vi "KI6221.vi"() -> ()   [LabVIEW 2019] (continued)
                n2609 = call "WriteToFile.vi"("character string"=w5028, "file path (dialog if empty)"=w4969) -> ("new file path (Not A Path if cancelled)"=w5027:path)  [unwired: 3 in]
                n2610 = Path To String(path=w5027) -> (string=w4971:string)
                n2611 = Equal?(x=w4972, y=w4971) -> (x = y?=w4970:bool)
                n2612 = call "CreateDataFiles.vi"("new file path (Not A Path if cancelled)"=w5025, "attachments"="attachments", "path"=w4969, "selection"=w4970, "DELTA DATASHEET"=w4974, "PULSE DATASHEET"=w4975, "DIFF CON DATASHEET"=w4976, "ATTACHMENTS"=w4977) -> ()
              }
              frame True {
              }
            }
          }
        }
        n2613 = control-ref of="Main Tabs"() -> (w156:refnum<vi>)
        n2614 = control-ref of="COMM\nTab Control"() -> (w189:refnum<vi>)
        n2615 = control-ref of="4 step TABS"() -> (w188:refnum<vi>)
        n2616 = control-ref of="Default path"() -> (w190:refnum<vi>)
        n2617 = local read "attachments"() -> (w186:T6)
        n2618 = local read "mail server"() -> (w187:string)
        n2619 = control-ref of="debug str"() -> (w173:refnum<vi>)
        n2620 = control-ref of="Main Tabs"() -> (w155:refnum<vi>)
        n2621 = call "WebUpdate.vi"("Settings Cluster"=w169, "WEB UPDATES"=FALSE, "Web Updates button"=w171, "Big Tabs"=w155, "Web Update String"=w170, "Default Path"=w172) -> ()  [unwired: 4 out]
        n2622 = call "KIBugReport.vi"("BUG REPORT"="BUG REPORT", "attachments"=w186, "mail server"=w187, "Big Tabs"=w155, "Debug Str"=w173) -> ("error out 6"=→"error out 6":errorcluster)  [unwired: 1 in]
        n2623 = Or(x="connect HELP LINK", y="connect HELP LINK 2") -> (x .or. y?=w167:bool)
        n2624 = call "WebLinks.vi"("Default Path"=w190, "Big Tabs"=w156, "4 step TABS"=w188, "COMM TABS"=w189, "ARB HELP LINK"=FALSE, "MAIN HELP LINK"="MAIN HELP LINK", "connect HELP LINK"=w167, "PULSE HELP LINK"="PULSE HELP LINK", "DC HELP LINK"="DC HELP LINK", "DELTA HELP LINK"="DELTA HELP LINK", "APPS"="APPS", "Guide help 3"="Guide help 3", "Guide help 2"="Guide help 2", "Guide help 1"="Guide help 1", "virtual front panel HELP LINK"="virtual front panel HELP LINK", "www"="www", "user's web"="user's web") -> ()  [unwired: 3 in]
        n2625 = local read "Setup String"() -> (w143:string)
        n2626 = local read "GPIB Array"() -> (w144:string[])
        n2627 = case shown="False" "Enable \nSTEP SOURCE" {
          frame False {
            w4628 = u8 2 ("Disabled")
            n2628 = property on="Start Level" class="DigNum (strict)"("Disabled"=w4628) -> ()  [unwired: 2 in, 2 out]
            n2629 = property on="Number of steps" class="DigNum (strict)"("Disabled"=w4628) -> ()  [unwired: 2 in, 2 out]
            n2630 = property on="Stop Level" class="DigNum (strict)"("Disabled"=w4628) -> ()  [unwired: 2 in, 2 out]
          }
          frame True {
            w4629 = u8 0 ("Disabled")
            n2631 = property on="Number of steps" class="DigNum (strict)"("Disabled"=w4629) -> ()  [unwired: 2 in, 2 out]
            n2632 = property on="Start Level" class="DigNum (strict)"("Disabled"=w4629) -> ()  [unwired: 2 in, 2 out]
            n2633 = property on="Stop Level" class="DigNum (strict)"("Disabled"=w4629) -> ()  [unwired: 2 in, 2 out]
          }
        }
        n2634 = local read "EXIT NOW"() -> (w192:bool)
        n2635 = Wait (ms)(milliseconds to wait=u32 100) -> ()  [unwired: 1 out]
        n2636 = call "Exit.vi"("EXIT 2"="EXIT 2") -> ("SAVE NOW"=w193:bool, "EXIT NOW"=w195:bool, "EXIT"=w194:bool)
        n2637 = call "ViewScpi.vi"("RUN ARB .H"="RUN ARB .H", "ABORT .H"="ABORT .H", "STOP ARB .H"="STOP ARB .H", "DATA .H"="DATA .H", "VIEW SCPI"="GENERATE SCPI - ADVANCED", "UPLOAD ARB .H"="UPLOAD ARB .H", "GPIB Array"=w144, "RUN DELTA .H"="RUN DELTA .H", "RUN DC .H"="RUN DC .H", "RUN PULSE .H"="RUN PULSE .H") -> ()
        n2638 = local write "EXIT 2"(w194) -> ()
        n2639 = local write "SAVE NOW"(w193) -> ()
        n2640 = local write "EXIT NOW"(w195) -> ()
        n2641 = call "ViewScpi-Basic2.vi"("SETUP STRING"=w143, "VIEW SCPI"="GENERATE SCPI - BASIC", "GPIB Array"=w144) -> ()  [unwired: 8 in]
        n2642 = local read "Select the interface for the 6220/6221:"() -> (w158:u16)
        n2643 = local read "VALID SETUP"() -> (w197:bool)
        n2644 = local read "SETUP YET?"() -> (w196:i32)
        n2645 = flat-sequence {
          tunnel: w200 -> [w4596]
          tunnel: [w4596] -> w201
          tunnel: w158 -> [w4599]
          tunnel: w201 -> [w4598]
          tunnel: [w4598] -> w199
          frame #0 {
            "6220 VISA" <- w4596
          }
          frame #1 {
            n2646 = case shown="True" "Case Constant\n(See Context Help) 8" {
              tunnel: w4599 -> [_ w4602]
              frame False {
              }
              frame True {
                n2647 = control-ref of="6220 VISA"() -> (w4601:refnum<vi>)
                n2648 = call "TcpipSetup.vi"("Model 6220 or 6221 is connected by:"=w4602, "reference"=w4601) -> ("error out"=→"error out 26":errorcluster)  [unwired: 1 in, 1 out]
              }
            }
          }
        }
        n2649 = Number To Decimal String(number="Select Network Card number:\n(default to zero)") -> (decimal integer string=w165:string)  [unwired: 1 in]
        n2650 = control-ref of=".  IP#2"() -> (w161:refnum<vi>)
        n2651 = call "VerifyText.vi"("SETUP YET?"=w196, "VALID SETUP"=w197) -> ("Text.TextColor"=w206:u32, "Value"=w207:string)
        n2652 = control-ref of="Input instrument IP Address:"() -> (w162:refnum<vi>)
        n2653 = control-ref of="Select GPIB Address number \nof the current source:"() -> (w163:refnum<vi>)
        n2654 = control-ref of=".  IP#4"() -> (w159:refnum<vi>)
        n2655 = control-ref of=".  IP#3"() -> (w160:refnum<vi>)
        n2656 = local read "GPIB Array"() -> (w176:string[])
        n2657 = property on="instrument status" class="Str"("Value"=w207, "Text.Text Colors:Text Color"=w206) -> ()  [unwired: 2 in, 2 out]
        n2658 = call "StepSrcVisaSetup.vi"("Value"="GPIB Address:", "Value 2"="Select GPIB Board number:\n(default to zero)") -> ("String"=w202:string, "String 2"=w203:string)
        "step VISA" <- w202
        n2659 = call "VisaString.vi"("IP 4"=w159, "NETwork card #"=w165, "IP 3"=w160, "IP 2"=w161, "GPIB addr"=w163, "IP 1"=w162, "GPIB board string"=w203, "Model 6220 or 6221 is connected by:"=w158) -> ("VISA string"=w200:string)
        n2660 = property on="demo warning" class="Str"("Visible"="DEMO MODE") -> ()  [unwired: 2 in, 2 out]
        n2661 = case shown="True" "Verify instruments" {
          tunnel: w199 -> [_ w4620]
          tunnel: w202 -> [_ w4619]
          tunnel: w176 -> [_ w4616]
          tunnel: [w4603 1 ("SETUP YET?")] -> w177
          frame False {
            n2662 = local read "SETUP YET?"() -> (w4603:i32)
          }
          frame True {
            w4608 = u8 0 ("Disabled")
            n2663 = property on="Select step source:" class="Ring (strict)"() -> ("Value"=w4617:u16, "Strings []"=w4618:string[])  [unwired: 2 in, 2 out]
            n2664 = property on="Verify instruments" class="Bool (strict)"("Disabled"=u8 2) -> ()  [unwired: 2 in, 2 out]
            n2665 = property on="Select the nanovoltmeter model number:" class="Ring (strict)"() -> ("Value"=w4622:u16)  [unwired: 2 in, 2 out]
            n2666 = property on="VERIFY:" class="Str"() -> ("Value"=w4614:string)  [unwired: 2 in, 2 out]
            n2667 = property on="Select the current source model number:" class="Ring (strict)"() -> ("Value"=w4623:u16)  [unwired: 2 in, 2 out]
            n2668 = property on="RESPONSE STRING:" class="Str"() -> ("Value"=w4613:string)  [unwired: 2 in, 2 out]
            n2669 = call "InstrVerify.vi"("Value 8"=w4623, "STEP SOURCE TEST"=FALSE ("Value 5"), "Value 2"=w4614, "Value"=w4613, "Value 3"=w4616, "Value 4"=w4617, "Value 7"=w4622, "Strings []"=w4618, "String"=w4619, "String 2"=w4620) -> ("Disabled"=w4625:u8, "Value 6"=w4610:bool, "error in (no error)"=w4621:errorcluster, "error"=→"error out 13":errorcluster, "Value 9"=w4626:bool, "error out"=→"error out 14":errorcluster)
            n2670 = property on="Verify instruments" class="Bool (strict)"(error in=w4621, "Disabled"=w4625) -> (error out=w4627:errorcluster)  [unwired: 1 in, 1 out]
            n2671 = property on="Verify instruments" class="Bool (strict)"(error in=w4627, "Value"=w4626) -> (error out=w4605:errorcluster)  [unwired: 1 in, 1 out]
            n2672 = local write "VALID SETUP"(w4610) -> ()
            n2673 = local write "NEXT FLAG LAST"(-1 ("NEXT FLAG LAST")) -> ()
            n2674 = property on="NEXT" class="Bool"(error in=w4605, "Disabled"=w4608) -> (error out=w4606:errorcluster)  [unwired: 1 in, 1 out]
            n2675 = property on="BACK" class="Bool"(error in=w4606, "Disabled"=w4608) -> (error out=→"error out 12":errorcluster)  [unwired: 1 in, 1 out]
          }
        }
        "SETUP YET?" <- w177
        n2676 = case shown="True" "OPEN" {
          frame False {
          }
          frame True {
            n2677 = property on="output cluster" class="Clust (strict)"() -> ("Value"=w4640:T10)  [unwired: 2 in, 2 out]
            n2678 = local read "FIRST OPEN"() -> (w4636:bool)
            n2679 = local read "Default path"() -> (w4637:path)
            n2680 = local write "OPEN"(FALSE) -> ()
            n2681 = call "DataFileNames.vi"("Default path"=w4637, "FIRST OPEN"=w4636, "Value 2"=w4640, "Current file"="") -> ("search string/char (-) 3"=w4643:string, "Value"=w4639:T15, "Path"=w4635:path, "CANCELLED"=w4632:bool, "search string/char (-) 2"=w4642:string, "err"=w4633:bool, "search string/char (-)"=w4641:string)
            n2682 = case shown="False" w4632 {
              tunnel: w4635 -> [w4647 _]
              tunnel: w4643 -> [w4651 _]
              tunnel: w4642 -> [w4650 _]
              tunnel: w4641 -> [w4649 _]
              tunnel: w4639 -> [w4648 _]
              tunnel: w4633 -> [w4646 _]
              frame False {
                n2683 = case shown="False" w4646 {
                  tunnel: w4651 -> [w4778 _]
                  tunnel: w4650 -> [w4777 _]
                  tunnel: w4649 -> [w4776 _]
                  tunnel: w4648 -> [w4723 _]
                  tunnel: w4647 -> [w4691 _]
                  frame False {
                    (unwired) dbl[][] array7x67001[469007 elements] ("array")
                    w4755 = -2 ("index")
                    w4692 = FALSE
                    n2684 = control-ref of="GPIB Address:"() -> (w4703:refnum<vi>)
                    n2685 = control-ref of="DELAY in mS"() -> (w4697:refnum<vi>)
                    n2686 = control-ref of="GO TO LEVEL:                *NOTE - MUST include <LEVEL>"() -> (w4704:refnum<vi>)
                    n2687 = control-ref of="INSTRUMENT NAME:"() -> (w4702:refnum<vi>)
                    n2688 = control-ref of="VERIFY:"() -> (w4701:refnum<vi>)
                    n2689 = control-ref of="RESPONSE STRING:"() -> (w4700:refnum<vi>)
                    n2690 = control-ref of="CONFIGURE:"() -> (w4699:refnum<vi>)
                    n2691 = control-ref of="DEACTIVATE:"() -> (w4698:refnum<vi>)
                    n2692 = control-ref of="MASTER DRIVER Array"() -> (w4696:refnum<vi>)
                    n2693 = control-ref of="Select step source:"() -> (w4705:refnum<vi>)
                    n2694 = control-ref of="Default path"() -> (w4695:refnum<vi>)
                    n2695 = control-ref of="Differential Conductance Surface Plot"() -> (w4713:refnum<vi>)
                    n2696 = control-ref of="Y AXIS LAST -PULSE"() -> (w4711:refnum<vi>)
                    n2697 = control-ref of="PULSE DATA SHEET"() -> (w4712:refnum<vi>)
                    n2698 = control-ref of="Differential Conductance Measurement Data"() -> (w4716:refnum<vi>)
                    n2699 = control-ref of="Y AXIS LAST -DELTA"() -> (w4709:refnum<vi>)
                    n2700 = control-ref of="Delta Mode Measurement Data"() -> (w4710:refnum<vi>)
                    n2701 = control-ref of="Pulsed IV Graph"() -> (w4707:refnum<vi>)
                    n2702 = control-ref of="Y AXIS LAST -DC"() -> (w4715:refnum<vi>)
                    n2703 = control-ref of="Differential Conductance Graph"() -> (w4714:refnum<vi>)
                    n2704 = control-ref of="Delta Mode Resistance Graph"() -> (w4708:refnum<vi>)
                    n2705 = local read "MASTER DRIVER Array"() -> (w4693:T9)
                    n2706 = local write "VALID SETUP"(w4692) -> ()
                    n2707 = local write "FIRST OPEN"(w4692) -> ()
                    n2708 = local write "SETUP YET?"(0 ("Numeric 2")) -> ()
                    n2709 = call "LoadSavedData.vi"("DCON DATA"=w4716, "search string/char (-)"=w4776, "search string/char (-) 2"=w4777, "Y axis last DCON"=w4715, "search string/char (-) 3"=w4778, "DCON 2d Graph"=w4714, "Path"=w4691, "DCON 3D plot"=w4713, "DELTA GRAPH"=w4708, "PULSE DATASHEET"=w4712, "x axis last pulse"=w4711, "PULSE GRAPH"=w4707, "DELTA DATASHEET"=w4710, "Y axis last DELTA"=w4709) -> ()  [unwired: 2 in]
                    n2710 = Unbundle(w4723) -> ("Value"=w4867:dbl, "Value"=w4866:i32, "Value"=w4865:u16, "Value"=w4864:bool, "Value"=w4863:dbl, "Value"=w4862:i32, "Value"=w4861:u16, "Value"=w4860:dbl, "Value"=w4859:dbl, "Value"=w4858:bool, "Value"=w4857:dbl, "Value"=w4856:dbl, "Value"=w4855:u16, "Value"=w4854:dbl, "Value"=w4853:dbl, "Value"=w4852:i32, "Value"=w4851:dbl, "Value"=w4850:dbl, "Value"=w4774:u16, "Value"=w4849:i32, "Value"=w4848:u16, "Value"=w4847:u16, "Value"=w4846:dbl, "Value"=w4845:dbl, "Value"=w4773:u16, "Value"=w4844:bool, "Value"=w4843:dbl, "Value"=w4842:i32, "Value"=w4841:i32, "Value"=w4840:u16, "Value"=w4839:dbl, "Value"=w4769:dbl, "Value"=w4838:u16, "Value"=w4837:dbl, "Value"=w4836:dbl, "Value"=w4835:dbl, "Value"=w4834:dbl, "Value"=w4833:u16, "Value"=w4771:dbl, "Value"=w4832:i32, "complete number of cycles"=w4775:dbl, "Value"=w4770:i32, "Value"=w4831:dbl, "Value"=w4830:dbl, "Value"=w4829:dbl, "Value"=w4828:dbl, "Value"=w4827:dbl, "Value"=w4826:u16, "Value"=w4825:dbl, "Value"=w4824:dbl, "Value"=w4823:dbl, "Value"=w4822:u16, "Value"=w4821:u16, "Value"=w4772:bool, "Value"=w4780:i32, "Value"=w4820:u16, "Value"=w4819:i32, "Value"=w4684:bool, "Value"=w4818:u16, "Value"=w4783:i32, "Value"=w4817:u16, "Value"=w4816:u16, "Value"=w4787:u16, "Value"=w4781:i32, "Value"=w4815:bool, "Value"=w4788:u16, "Value"=w4782:i32, "Value"=w4779:i32, "Value"=w4814:bool, "Value"=w4813:i32, "result string"=w4811:string, "result string"=w4810:string, "result string"=w4809:string, "result string"=w4808:string, "result string"=w4807:string, "result string"=w4806:string, "Value"=w4802:i32, "Value"=w4803:i32, "Value"=w4812:bool, "String"=w4804:string, "PULSE - SWEEP #STEPS"=w4767:i32, "Sawtooth NUM CYCLES"=w4734:dbl, "Sawtooth Offset (Amps) 2"=w4735:dbl, "Duty Cycle (%) 2"=w4736:dbl, "Start Phase \n(Degrees) 2"=w4737:dbl, "SQUARE Number of Points per cycle 2"=w4738:i32, "SQUARE Number of Cycles 2"=w4739:dbl, "SQUARE Amplitude (Amps) 2"=w4740:dbl, "SQUARE Offset (Amps) 2"=w4741:dbl, "SQUARE Duty Cycle (%) 3"=w4742:dbl, "SQUARE Start Phase \n(Degrees) 3"=w4743:dbl, "SQUARE Rise/Fall in points 2"=w4744:i32, "SINE Number of Points per cycle 2"=w4745:i32, "SINE Number of Cycles 2"=w4746:dbl, "SINE Amplitude (Amps) 2"=w4747:dbl, "SINE Offset (Amps) 2"=w4748:dbl, "SINE Start Phase \n(Degrees) 3"=w4749:dbl, "NOISE Number of Points per cycle 2"=w4750:i32, "NOISE Number of Cycles 2"=w4751:dbl, "NOISE Standard Deviation 2"=w4752:dbl, "NOISE Offset (Amps) 2"=w4753:dbl, "Analog filter - \nTau in # points 2"=w4754:dbl, "ScratchPad Array 2"=w4659:dbl[][], "ScratchPad Array Cnt 2"=w4657:i32[], "Item Names"=w4725:string[], "ADD 5"=w4724:i32[], "Complete Array 2"=w4731:dbl[][], "Complete Array Cnt 2"=w4732:i32[], "Item Names 5"=w4726:string[], "ADD 7"=w4727:i32[], "waveform holder 2"=w4733:dbl[], "ADD 6"=w4730:i32[], "ADD 8"=w4729:i32[], "ADD 9"=w4728:i32[], "Trace offset (% Pk-Pk): 2"=w4722:dbl, "phase enable 2"=w4718:bool, "Phase Value 2"=w4719:dbl, "triggerline 2"=w4720:i16, "Pulse Off Level (Amps) 2"=w4721:dbl, "ARB VOLT COMP"=w4717:dbl, "nV CAP"=w4686:u16, "Pulse Filter 2"=w4690:u16, "Pulse FIlter Count 2"=w4689:i32, "Setup String"=w4688:string, "DCON filter state"=w4687:u16, "Source Level (Amps) 3"=w4683:dbl, "Current Source \nVoltage Compliance (V) 4"=w4682:dbl, "Start Current (Amps) 3"=w4681:dbl, "Stop Current (Amps) 3"=w4680:dbl, "Number of sweep points 3"=w4679:i32, "Sweep Type 3"=w4678:u16, "Current Source \nVoltage Compliance (V) 5"=w4677:dbl, "Delay (settle time in sec) 3"=w4676:dbl, "enable measure 3"=w4675:bool, "Voltage Measure Range 3"=w4674:dbl, "Measurement Integration \n(NPLCs) 3"=w4673:dbl, "Waveform Type  3"=w4672:u16, "I Sweep V Measure Data 3"=w4671:string[][], "Ramp from: (Amps) 3"=w4670:dbl, "Ramp to: (Amps) 3"=w4669:dbl, "Duty Cycle (%) 4"=w4668:dbl, "Amplitude (Amps) 4"=w4667:dbl, "Offset (Amps) 4"=w4666:dbl, "Duty Cycle (%) 5"=w4665:dbl, "Amplitude (Amps) 5"=w4664:dbl, "Offset (Amps) 5"=w4663:dbl, "Signal Repetition \nFrequency (Hz) 3"=w4662:dbl, "Voltage\n Compliance3"=w4661:dbl, "Number of Zero Measurements 2"=w4660:i32)
                    n2711 = local write "Setup String"(w4688) -> ()
                    n2712 = property on="ARB\nVoltage\n Compliance" class="DigNum (strict)"("Value"=w4717) -> ()  [unwired: 2 in, 2 out]
                    n2713 = Array Size(array=w4657) -> (size(s)=w4654:i32)
                    n2714 = property on="DELAY in mS" class="DigNum (strict)"("Value"=w4802) -> ()  [unwired: 2 in, 2 out]
                    n2715 = Initialize Array(0.0 ("element"), w4654, 66000 ("dimension size")) -> (w4652:dbl[][])
                    n2716 = property on="GPIB Address:" class="DigNum (strict)"("Value"=w4803) -> ()  [unwired: 2 in, 2 out]
                    n2717 = property on="Pulse Off Level (Amps)" class="DigNum (strict)"("Value"=w4721) -> ()  [unwired: 2 in, 2 out]
                    n2718 = property on="Trace offset (% Pk-Pk):" class="DigNum (strict)"("Value"=w4722) -> ()  [unwired: 2 in, 2 out]
                    n2719 = property on="triggerline" class="DigNum (strict)"("Value"=w4720) -> ()  [unwired: 2 in, 2 out]
                    n2720 = property on="phase enable" class="Bool (strict)"("Value"=w4718) -> ()  [unwired: 2 in, 2 out]
                    n2721 = property on="Complete Waveform" class="LstBox (strict)"("Item Names"=w4726, "Value"=w4727) -> (error out=w4766:errorcluster)  [unwired: 2 in, 1 out]
                    n2722 = property on="waveform holder" class="Arr (strict)"(error in=w4766, "Value"=w4733) -> (error out=w4765:errorcluster)  [unwired: 1 in, 1 out]
                    n2723 = property on="Complete Array" class="Arr (strict)"(error in=w4765, "Value"=w4731) -> (error out=w4764:errorcluster)  [unwired: 1 in, 1 out]
                    n2724 = property on="Complete Array Cnt" class="Arr (strict)"(error in=w4764, "Value"=w4732) -> (error out=w4763:errorcluster)  [unwired: 1 in, 1 out]
                    n2725 = property on="ScratchPad" class="LstBox (strict)"(error in=w4763, "Item Names"=w4725, "Value"=w4724) -> (error out=w4762:errorcluster)  [unwired: 1 in, 1 out]
                    n2726 = property on="ADD 2" class="LstBox (strict)"(error in=w4762, "Item Names"=w4725, "Value"=w4729) -> (error out=w4761:errorcluster)  [unwired: 1 in, 1 out]
                    n2727 = property on="ADD" class="LstBox (strict)"(error in=w4761, "Item Names"=w4725, "Value"=w4730) -> (error out=w4760:errorcluster)  [unwired: 1 in, 1 out]
                    n2728 = property on="filter" class="LstBox (strict)"(error in=w4760, "Item Names"=w4725, "Value"=w4728) -> (error out=w4759:errorcluster)  [unwired: 1 in, 1 out]
                    n2729 = property on="ScratchPad Array Cnt" class="Arr (strict)"(error in=w4759, "Value"=w4657) -> (error out=w4758:errorcluster)  [unwired: 1 in, 1 out]
                    n2730 = property on="INFINITE REPEAT PULSE CYCLES" class="Bool (strict)"("Value"=w4812) -> ()  [unwired: 2 in, 2 out]
                    n2731 = property on="Phase Value" class="DigNum (strict)"("Value"=w4719) -> ()  [unwired: 2 in, 2 out]
                    n2732 = call "StepSrcFileOpen.vi"("result string 2"=w4807, "result string 3"=w4808, "result string 4"=w4809, "result string 5"=w4810, "result string 6"=w4811, "MASTER DRIVER Array"=w4693, "result string"=w4806, "Value 7"=w4802, "Value 8"=w4803, "String"=w4804) -> ("Value 9"=w4805:string, "Value 3"=w4798:string, "Value 6"=w4801:string, "Value"=w4768:string, "Boolean"=w4795:bool, "Numeric"=w4794:i32, "Boolean 2"=w4796:bool, "Value 2"=w4797:string, "Value 4"=w4799:string, "Value 5"=w4800:string)
                    n2733 = property on="INSTRUMENT NAME:" class="Str"("Value"=w4768) -> ()  [unwired: 2 in, 2 out]
                    n2734 = property on="GO TO LEVEL:                *NOTE - MUST include <LEVEL>" class="Str"("Value"=w4798) -> ()  [unwired: 2 in, 2 out]
                    n2735 = property on="CONFIGURE:" class="Str"("Value"=w4799) -> ()  [unwired: 2 in, 2 out]
                    n2736 = property on="VERIFY:" class="Str"("Value"=w4801) -> ()  [unwired: 2 in, 2 out]
                    n2737 = call "LoadStepSrc.vi"("reference"=w4705, "Boolean"=w4795, "Numeric"=w4794, "reference 2"=w4704, "Boolean 2"=w4796, "reference 3"=w4703, "reference 11"=w4695, "reference 4"=w4702, "reference 10"=w4696, "reference 5"=w4701, "reference 6"=w4700, "reference 7"=w4699, "reference 8"=w4698, "reference 9"=w4697) -> ("error out 34"=→"error out 34":errorcluster)  [unwired: 1 in]
                    n2738 = property on="Test file description and comments:" class="Str"("Value"=w4805) -> ()  [unwired: 2 in, 2 out]
                    n2739 = property on="DEACTIVATE:" class="Str"("Value"=w4797) -> ()  [unwired: 2 in, 2 out]
                    n2740 = property on="RESPONSE STRING:" class="Str"("Value"=w4800) -> ()  [unwired: 2 in, 2 out]
                    n2741 = Insert Into Array(array=w4652, index (col)=0 ("index (row)"), new element=w4659) -> (w4658:dbl[][])  [unwired: 1 in]
                    n2742 = property on="ScratchPad Array" class="Arr (strict)"(error in=w4758, "Value"=w4658) -> (error out=w4756:errorcluster)  [unwired: 1 in, 1 out]
                    n2743 = property on="Pad Last" class="DigNum (strict)"(error in=w4756, "Value"=w4755) -> (error out=w4757:errorcluster)  [unwired: 1 in, 1 out]
                    n2744 = property on="Graph Last" class="DigNum (strict)"(error in=w4757, "Value"=w4755) -> ()  [unwired: 1 in, 2 out]
                    n2745 = property on="Number of Pulses" class="DigNum (strict)"("Value"=w4767) -> ()  [unwired: 2 in, 2 out]
                    n2746 = local write "Current Source \nVoltage Compliance (V)"(w4682) -> ()
                    n2747 = local write "Current Source \nVoltage Compliance (V)"(w4677) -> ()
                    n2748 = local write "Measurement Integration \n(NPLCs)"(w4673) -> ()
                    n2749 = local write "Number of sweep points"(w4679) -> ()
                    n2750 = local write "Delay (settle time in sec)"(w4676) -> ()
                    n2751 = local write "Source Level (Amps)"(w4683) -> ()
                    n2752 = local write "Start Current (Amps)"(w4681) -> ()
                    n2753 = local write "Stop Current (Amps)"(w4680) -> ()
                    n2754 = local write "Voltage Measure Range"(w4674) -> ()
                    n2755 = local write "I Sweep V Measure Data"(w4671) -> ()
                    n2756 = local write "enable measure"(w4675) -> ()
                    n2757 = local write "Waveform Type"(w4672) -> ()
                    n2758 = local write "Sweep Type"(w4678) -> ()
                    n2759 = property on="High Current (Amps)" class="DigNum (strict)"("Value"=w4867) -> ()  [unwired: 2 in, 2 out]
                    n2760 = property on="INFINITE DELTA CYCLES" class="Bool (strict)"("Value"=w4864) -> ()  [unwired: 2 in, 2 out]
                    n2761 = property on="Y Axis:" class="Ring (strict)"("Value"=w4861) -> ()  [unwired: 2 in, 2 out]
                    n2762 = property on="DAMPING" class="Bool (strict)"("Value"=w4858) -> ()  [unwired: 2 in, 2 out]
                    n2763 = property on="X Axis:" class="Ring (strict)"("Value"=w4855) -> ()  [unwired: 2 in, 2 out]
                    n2764 = property on="Start Current (Amps)" class="DigNum (strict)"("Value"=w4853) -> ()  [unwired: 2 in, 2 out]
                    n2765 = property on="Stop Current (Amps)" class="DigNum (strict)"("Value"=w4850) -> ()  [unwired: 2 in, 2 out]
                    n2766 = property on="I want to control my test in terms of:" class="Ring (strict)"("Value"=w4848) -> ()  [unwired: 2 in, 2 out]
                    n2767 = property on="Start Level" class="DigNum (strict)"("Value"=w4845) -> ()  [unwired: 2 in, 2 out]
                    n2768 = property on="Stop Level" class="DigNum (strict)"("Value"=w4843) -> ()  [unwired: 2 in, 2 out]
                    n2769 = property on="Horizontal Axis:" class="Ring (strict)"("Value"=w4838) -> ()  [unwired: 2 in, 2 out]
                    n2770 = property on="Resistance in Ohms" class="DigNum (strict)"("Value"=w4835) -> ()  [unwired: 2 in, 2 out]
                    n2771 = property on=".  IP#2" class="DigNum (strict)"("Value"=w4780) -> ()  [unwired: 2 in, 2 out]
                    n2772 = property on="X Axis:" class="Ring (strict)"("Value"=w4833) -> ()  [unwired: 2 in, 2 out]
                    n2773 = property on="Stop Pulse Level (Amps)" class="DigNum (strict)"("Value"=w4830) -> ()  [unwired: 2 in, 2 out]
                    n2774 = property on="Start Pulse Level (Amps)" class="DigNum (strict)"("Value"=w4827) -> ()  [unwired: 2 in, 2 out]
                    n2775 = property on="Interval between Pulses (NPLC)" class="DigNum (strict)"("Value"=w4824) -> ()  [unwired: 2 in, 2 out]
                    n2776 = property on="Pulse Mode:" class="Ring (strict)"("Value"=w4821) -> ()  [unwired: 2 in, 2 out]
                    n2777 = property on="Vertical Axis:" class="Ring (strict)"("Value"=w4840) -> ()  [unwired: 2 in, 2 out]
                    n2778 = local write "CAP IN"(w4686) -> ()
                    n2779 = property on="LOW to EARTH" class="Bool (strict)"("Value"=w4684) -> ()  [unwired: 2 in, 2 out]
                    n2780 = property on="Select the nanovoltmeter model number:" class="Ring (strict)"("Value"=w4820) -> ()  [unwired: 2 in, 2 out]
                    n2781 = property on="6220 Connect" class="Ring (strict)"("Value"=w4818) -> ()  [unwired: 2 in, 2 out]
                    n2782 = property on="HI IMP devices?" class="Ring (strict)"("Value"=w4816) -> ()  [unwired: 2 in, 2 out]
                    n2783 = property on="Pulse Level (Amps)" class="DigNum (strict)"("Value"=w4829) -> ()  [unwired: 2 in, 2 out]
                    n2784 = property on="Y Axis:" class="Ring (strict)"("Value"=w4826) -> ()  [unwired: 2 in, 2 out]
                    n2785 = property on="Current Source \nVoltage Compliance (V)" class="DigNum (strict)"("Value"=w4823) -> ()  [unwired: 2 in, 2 out]
                    n2786 = property on="Filter\nCount" class="DigNum (strict)"("Value"=w4866) -> ()  [unwired: 2 in, 2 out]
                    n2787 = property on="Low Current (Amps)" class="DigNum (strict)"("Value"=w4863) -> ()  [unwired: 2 in, 2 out]
                    n2788 = property on="Delay (mS) - settle time" class="DigNum (strict)"("Value"=w4860) -> ()  [unwired: 2 in, 2 out]
                    n2789 = property on="Measurement Integration (NPLCs)" class="DigNum (strict)"("Value"=w4857) -> ()  [unwired: 2 in, 2 out]
                    n2790 = property on="Current Source Range" class="Ring (strict)"("Value"=w4854) -> ()  [unwired: 2 in, 2 out]
                    n2791 = local write "FILTER"(w4687) -> ()
                    n2792 = property on="Number of sweep points" class="DigNum (strict)"("Value"=w4852) -> ()  [unwired: 2 in, 2 out]
                    n2793 = property on="Define source points with an:" class="Ring (strict)"("Value"=w4847) -> ()  [unwired: 2 in, 2 out]
                    n2794 = property on="Number of steps" class="DigNum (strict)"("Value"=w4842) -> ()  [unwired: 2 in, 2 out]
                    n2795 = property on="Voltage Measure Range" class="Ring (strict)"("Value"=w4839) -> ()  [unwired: 2 in, 2 out]
                    n2796 = property on="Current Source \nVoltage Compliance (V)" class="DigNum (strict)"("Value"=w4837) -> ()  [unwired: 2 in, 2 out]
                    n2797 = property on="Stop Voltage (Volts)" class="DigNum (strict)"("Value"=w4834) -> ()  [unwired: 2 in, 2 out]
                    n2798 = property on="Waveform Type" class="Ring (strict)"("Value"=w4774) -> ()  [unwired: 2 in, 2 out]
                    n2799 = property on="INF" class="Bool (strict)"("Value"=w4772) -> ()  [unwired: 2 in, 2 out]
                    n2800 = property on="Total Wave Duration (S)" class="DigNum (strict)"("Value"=w4775) -> ()  [unwired: 2 in, 2 out]
                    n2801 = property on="Signal Repetition \nFrequency (Hz)" class="DigNum (strict)"("Value"=w4771) -> ()  [unwired: 2 in, 2 out]
                    n2802 = property on="Graph view:" class="Ring (strict)"("Value"=w4773) -> ()  [unwired: 2 in, 2 out]
                    n2803 = property on="Power:" class="Ring (strict)"("Value"=w4817) -> ()  [unwired: 2 in, 2 out]
                    n2804 = local write "Pulse Filter Count"(w4689) -> ()
                    n2805 = local write "PULSE FILTER"(w4690) -> ()
                    n2806 = property on="FILTER" class="Ring (strict)"("Value"=w4865) -> ()  [unwired: 2 in, 2 out]
                    n2807 = property on="Number of Readings" class="DigNum (strict)"("Value"=w4862) -> ()  [unwired: 2 in, 2 out]
                    n2808 = property on="Voltage Measure Range" class="Ring (strict)"("Value"=w4859) -> ()  [unwired: 2 in, 2 out]
                    n2809 = property on="Current Source \nVoltage Compliance (V)" class="DigNum (strict)"("Value"=w4856) -> ()  [unwired: 2 in, 2 out]
                    n2810 = property on="Start Voltage  (Volts)" class="DigNum (strict)"("Value"=w4851) -> ()  [unwired: 2 in, 2 out]
                    n2811 = property on="Delay (settle time in mS)" class="DigNum (strict)"("Value"=w4846) -> ()  [unwired: 2 in, 2 out]
                    n2812 = property on="DIFF COND DAMPING" class="Bool (strict)"("Value"=w4844) -> ()  [unwired: 2 in, 2 out]
                    n2813 = property on="Repeat Filter Count:" class="DigNum (strict)"("Value"=w4841) -> ()  [unwired: 2 in, 2 out]
                    n2814 = property on="Measurement Integration (NPLCs)" class="DigNum (strict)"("Value"=w4836) -> ()  [unwired: 2 in, 2 out]
                    n2815 = property on="Number of Readings" class="DigNum (strict)"("Value"=w4832) -> ()  [unwired: 2 in, 2 out]
                    n2816 = property on="Delay - pulse settle time in mS" class="DigNum (strict)"("Value"=w4831) -> ()  [unwired: 2 in, 2 out]
                    n2817 = property on="Voltage Measure Range" class="Ring (strict)"("Value"=w4828) -> ()  [unwired: 2 in, 2 out]
                    n2818 = property on="Pulse Width (mS)" class="DigNum (strict)"("Value"=w4825) -> ()  [unwired: 2 in, 2 out]
                    n2819 = property on="Sweep Type" class="Ring (strict)"("Value"=w4822) -> ()  [unwired: 2 in, 2 out]
                    n2820 = property on="Number of sweep points" class="DigNum (strict)"("Value"=w4849) -> ()  [unwired: 2 in, 2 out]
                    n2821 = property on="Select Network Card number:\n(default to zero)" class="DigNum (strict)"("Value"=w4819) -> ()  [unwired: 2 in, 2 out]
                    n2822 = property on="Input instrument IP Address:" class="DigNum (strict)"("Value"=w4783) -> ()  [unwired: 2 in, 2 out]
                    n2823 = property on="Ramp from: (Amps)" class="DigNum (strict)"("Value"=w4769) -> ()  [unwired: 2 in, 2 out]
                    n2824 = property on="Select the current source model number:" class="Ring (strict)"("Value"=w4788) -> ()  [unwired: 2 in, 2 out]
                    n2825 = property on="Select the interface for the 6220/6221:" class="Ring (strict)"("Value"=w4787) -> ()  [unwired: 2 in, 2 out]
                    n2826 = local write "Number of Pulse Off Measurements"(w4660) -> ()
                    n2827 = property on="Number of Cycles" class="DigNum (strict)"("Value"=w4734) -> ()  [unwired: 2 in, 2 out]
                    n2828 = property on="Ramp to: (Amps)" class="DigNum (strict)"("Value"=w4735) -> ()  [unwired: 2 in, 2 out]
                    n2829 = property on="Duty Cycle (%)" class="DigNum (strict)"("Value"=w4736) -> ()  [unwired: 2 in, 2 out]
                    n2830 = property on="Start Phase \n(Degrees)" class="DigNum (strict)"("Value"=w4737) -> ()  [unwired: 2 in, 2 out]
                    n2831 = property on="Number of Points per cycle" class="DigNum (strict)"("Value"=w4738) -> ()  [unwired: 2 in, 2 out]
                    n2832 = property on="Number of Cycles" class="DigNum (strict)"("Value"=w4739) -> ()  [unwired: 2 in, 2 out]
                    n2833 = property on="Amplitude (Amps)" class="DigNum (strict)"("Value"=w4740) -> ()  [unwired: 2 in, 2 out]
                    n2834 = property on="Offset (Amps)" class="DigNum (strict)"("Value"=w4741) -> ()  [unwired: 2 in, 2 out]
                    n2835 = property on="Duty Cycle (%)" class="DigNum (strict)"("Value"=w4742) -> ()  [unwired: 2 in, 2 out]
                    n2836 = property on="Start Phase \n(Degrees)" class="DigNum (strict)"("Value"=w4743) -> ()  [unwired: 2 in, 2 out]
                    n2837 = property on="Rise/Fall in points" class="DigNum (strict)"("Value"=w4744) -> ()  [unwired: 2 in, 2 out]
                    n2838 = local write "Signal Repetition \nFrequency (Hz)"(w4662) -> ()
                    n2839 = local write "Voltage\n Compliance"(w4661) -> ()
                    n2840 = local write "Ramp from: (Amps)"(w4670) -> ()
                    n2841 = local write "Amplitude (Amps)"(w4667) -> ()
                    n2842 = local write "Amplitude (Amps)"(w4664) -> ()
                    n2843 = local write "Ramp to: (Amps)"(w4669) -> ()
                    n2844 = local write "Offset (Amps)"(w4666) -> ()
                    n2845 = local write "Offset (Amps)"(w4663) -> ()
                    n2846 = local write "Duty Cycle (%)"(w4668) -> ()
                    n2847 = local write "Duty Cycle (%)"(w4665) -> ()
                    n2848 = property on="Number of Points per cycle" class="DigNum (strict)"("Value"=w4770) -> ()  [unwired: 2 in, 2 out]
                    n2849 = Boolean To (0,1)(Boolean=w4684) -> (0, 1=w4685:i16)
                    n2850 = Equal?(x=1, y=w4788) -> (x = y?=w4789:bool)
                    n2851 = Equal?(x=2, y=w4787) -> (x = y?=w4790:bool)
                    n2852 = Or(x=w4789, y=w4790) -> (x .or. y?=w4791:bool)
                    n2853 = property on=".  IP#4" class="DigNum (strict)"("Value"=w4782) -> ()  [unwired: 2 in, 2 out]
                    n2854 = case shown="False" w4791 {
                      tunnel: [FALSE TRUE] -> w4786
                      tunnel: [TRUE FALSE] -> w4785
                      tunnel: [0 1] -> w4784
                      frame False {
                      }
                      frame True {
                        # "GPIB"
                      }
                    }
                    n2855 = property on="at GPIB Address:" class="DigNum (strict)"("Value"=w4779, "Visible"=w4786) -> ()  [unwired: 2 in, 2 out]
                    n2856 = local write "LOW to EARTH 2"(w4685) -> ()
                    n2857 = property on="DEFAULT setup" class="Bool (strict)"("Value"=w4814) -> ()  [unwired: 2 in, 2 out]
                    n2858 = property on="Select GPIB Address number \nof the current source:" class="DigNum (strict)"("Value"=w4779) -> ()  [unwired: 2 in, 2 out]
                    n2859 = property on=".  IP#3" class="DigNum (strict)"("Value"=w4781) -> ()  [unwired: 2 in, 2 out]
                    n2860 = property on="Number of Points per cycle" class="DigNum (strict)"("Value"=w4745) -> ()  [unwired: 2 in, 2 out]
                    n2861 = property on="Number of Cycles" class="DigNum (strict)"("Value"=w4746) -> ()  [unwired: 2 in, 2 out]
                    n2862 = property on="Amplitude (Amps)" class="DigNum (strict)"("Value"=w4747) -> ()  [unwired: 2 in, 2 out]
                    n2863 = property on="Offset (Amps)" class="DigNum (strict)"("Value"=w4748) -> ()  [unwired: 2 in, 2 out]
                    n2864 = property on="Start Phase \n(Degrees)" class="DigNum (strict)"("Value"=w4749) -> ()  [unwired: 2 in, 2 out]
                    n2865 = property on="Number of Points per cycle" class="DigNum (strict)"("Value"=w4750) -> ()  [unwired: 2 in, 2 out]
                    n2866 = property on="Number of Cycles" class="DigNum (strict)"("Value"=w4751) -> ()  [unwired: 2 in, 2 out]
                    n2867 = property on="Standard Deviation" class="DigNum (strict)"("Value"=w4752) -> ()  [unwired: 2 in, 2 out]
                    n2868 = property on="Offset (Amps)" class="DigNum (strict)"("Value"=w4753) -> ()  [unwired: 2 in, 2 out]
                    n2869 = property on="Analog filter - \nTau in # points" class="DigNum (strict)"("Value"=w4754) -> ()  [unwired: 2 in, 2 out]
                    n2870 = property on="Model 6220 or 6221 is connected by:" class="Ring (strict)"("Value"=w4784) -> ()  [unwired: 2 in, 2 out]
                    n2871 = property on="at instrument IP Address:" class="DigNum (strict)"("Value"=w4783, "Visible"=w4785) -> ()  [unwired: 2 in, 2 out]
                    n2872 = property on=".  IP#2" class="DigNum (strict)"("Value"=w4780, "Visible"=w4785) -> ()  [unwired: 2 in, 2 out]
                    n2873 = property on="Select GPIB Board number:\n(default to zero)" class="DigNum (strict)"("Value"=w4813) -> ()  [unwired: 2 in, 2 out]
                    n2874 = property on=".  IP#4" class="DigNum (strict)"("Value"=w4782, "Visible"=w4785) -> ()  [unwired: 2 in, 2 out]
                    n2875 = property on="Enable \nSTEP SOURCE" class="Bool (strict)"("Value"=w4815) -> ()  [unwired: 2 in, 2 out]
                    n2876 = property on=".  IP#3 2" class="DigNum (strict)"("Value"=w4781, "Visible"=w4785) -> ()  [unwired: 2 in, 2 out]
                  }
                  frame True {
                    n2877 = call "Saved Data file error"() -> ()  [unwired: 10 in, 2 out]
                  }
                }
              }
              frame True {
              }
            }
            n2878 = Or(x=w4632, y=w4636) -> (x .or. y?=w4634:bool)
            n2879 = case shown="False" w4634 {
              tunnel: [w4644 path ""] -> w4630
              tunnel: w4635 -> [w4644 _]
              frame False {
              }
              frame True {
              }
            }
            "Current Test File:" <- w4630
          }
        }
        n2880 = local read "Source TABS LAST"() -> (w154:u32)
        n2881 = local read "Main Tabs"() -> (w153:T1)
        n2882 = Not Equal?(x=w154, y=w148) -> (x != y?=w151:bool)
        n2883 = Not Equal?(x=w153, y=T1."Basic Operation" ("Big Tabs")) -> (x != y?=w150:bool)
        n2884 = And(x=w151, y=w150) -> (x .and. y?=w149:bool)
        n2885 = case shown="False" w149 {
          tunnel: w148 -> [_ w232]
          frame False {
          }
          frame True {
            n2886 = local write "Source TABS LAST"(w232) -> ()
          }
        }
      }
    }
    frame #5 {
      n2887 = case shown="True" "Case Constant\n(See Context Help) 9" {
        frame False {
        }
        frame True {
          n2888 = Current VI's Path() -> (path=w5060:path)
          n2889 = Open VI Reference(vi path=w5060) -> (vi reference=w5063:refnum<vi>, error out=w5062:errorcluster)  [unwired: 5 in]
          n2890 = invoke class="VI" method="FP.Close"(reference=w5063, error in=w5062) -> (error out=→"error out":errorcluster)  [unwired: 1 in, 2 out]
        }
      }
    }
  }
  n2891 = control-ref of="Default Cluster"() -> ()  [unwired: 1 out]
